vi "CAN react.vi"(4 "error in (no error)":errorcluster, 5 "Data":u8[](array[numeric]), 6 "COB id":i32, 7 "CANopen in":refnum<class "CANopen.lvclass">) -> (0 "error out":errorcluster, 3 "CANopen out":refnum<class "CANopen.lvclass">)   [LabVIEW 2024, in "canopen.lvlib" / "CANopen.lvclass"]
doc: "Starts the task that reads messages and tries to handle them."
uses:
  CANopen.lvclass
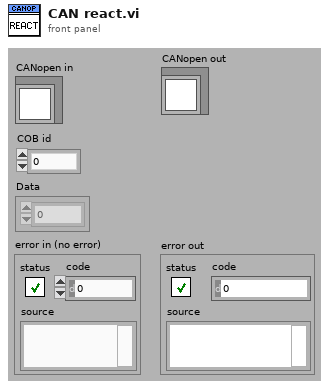
[diagram p1: front panel]
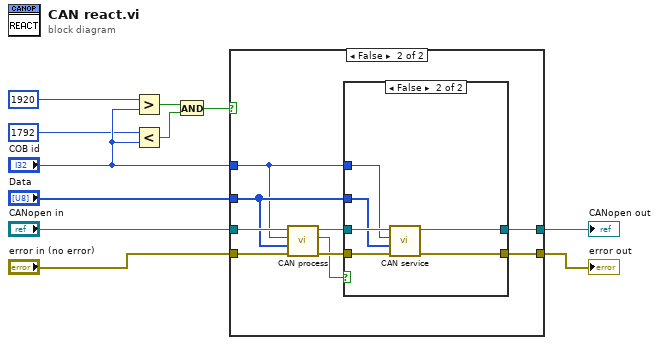
[diagram p0: block diagram]
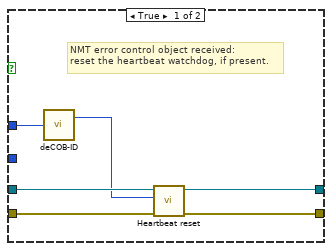
[diagram p2: hidden frame]
diagram:
  n1 = Greater?(x=1920, y="COB id") -> (0:w3:bool)
  n2 = Less?(x=1792, y="COB id") -> (x < y?=w2:bool)
  n3 = And(x=w3, y=w2) -> (x .and. y?=w1:bool)
  n4 = case shown="False" w1 {
    tunnel: "CANopen in" -> [w16 w23]
    tunnel: "error in (no error)" -> [w15 w22]
    tunnel: "Data" -> [_ w21]
    tunnel: [w14 w20] -> w8
    tunnel: [w13 w19] -> w7
    tunnel: "COB id" -> [w17 w18]
    frame True {
      # "NMT error control object received:\nreset the heartbeat watchdog, if present."
      n5 = call "deCOB-ID.vi"("Cob ID"=w17) -> ("Node ID"=w12:u16)  [unwired: 1 out]
      n6 = call "Heartbeat reset.vi"("error in"=w15, "Node ID"=w12, "CANopen in"=w16) -> ("error out"=w13:errorcluster, "CANopen out"=w14:refnum<class "CANopen.lvclass">)  [unwired: 3 out]
    }
    frame False {
      n7 = call "CAN process.vi"("error in (no error)"=w22, "Data"=w21, "COB id"=w18, "CANopen in"=w23) -> ("error out"=w26:errorcluster, "Processed?"=w25:bool, "CANopen out"=w24:refnum<class "CANopen.lvclass">)  [unwired: 1 out]
      n8 = case shown="False" w25 {
        tunnel: w26 -> [w28 w34]
        tunnel: [w28 w33] -> w19
        tunnel: [w27 w32] -> w20
        tunnel: w24 -> [w27 w31]
        tunnel: w18 -> [_ w30]
        tunnel: w21 -> [_ w29]
        frame True {
        }
        frame False {
          n9 = call "CAN service.vi"("error in (no error)"=w34, "Data"=w29, "COB id"=w30, "CANopen in"=w31) -> ("error out"=w33:errorcluster, "CANopen out"=w32:refnum<class "CANopen.lvclass">)  [unwired: 2 out]
        }
      }
    }
  }
  "CANopen out" <- w8
  "error out" <- w7
